vi "TimeOutPopUp.vi"(0 "Enable":bool=TRUE, 5 "error in (no error)":errorcluster, 7 "Timeout(s)":i32=2, 8 "Input Message":string="I am a Message" caption="String", 9 "Two Buttons?":bool=TRUE, 11 "Button Name":string="OK", 13 "Second Button Name":string="Cancel") -> (17 "Input":string, 18 "OK":bool, 19 "error out":errorcluster)   [LabVIEW 2018]
doc: "Displays a standard dialog box that prompts users to enter information, such as a user name and password.\n--------------------\n\nThis Express VI is configured as follows:\n\nMessage to Display to the User:I am a Message\nThe inputs are: \nText Entry Box: Input"
panel:
  out "min":dbl
  out "sec":dbl
  out "Position:Left Cancel":i32
  out "Position:Left OK1":i32
  out "Position:Top":i32
  out "Position:Left":i32
  in  "Cancel":bool
  in  "OK2":bool
  out "String":string="I am a Message" caption="There is no S11 Frequency Match. Check the Calibration and Frequency List.\nAlso Check the Frequency Units Match.\nThe test will automatically Start in 0 min 10 sec"
  in  "OK1":bool
  in  "Input 2":string caption="Input"
  out "REF":i32
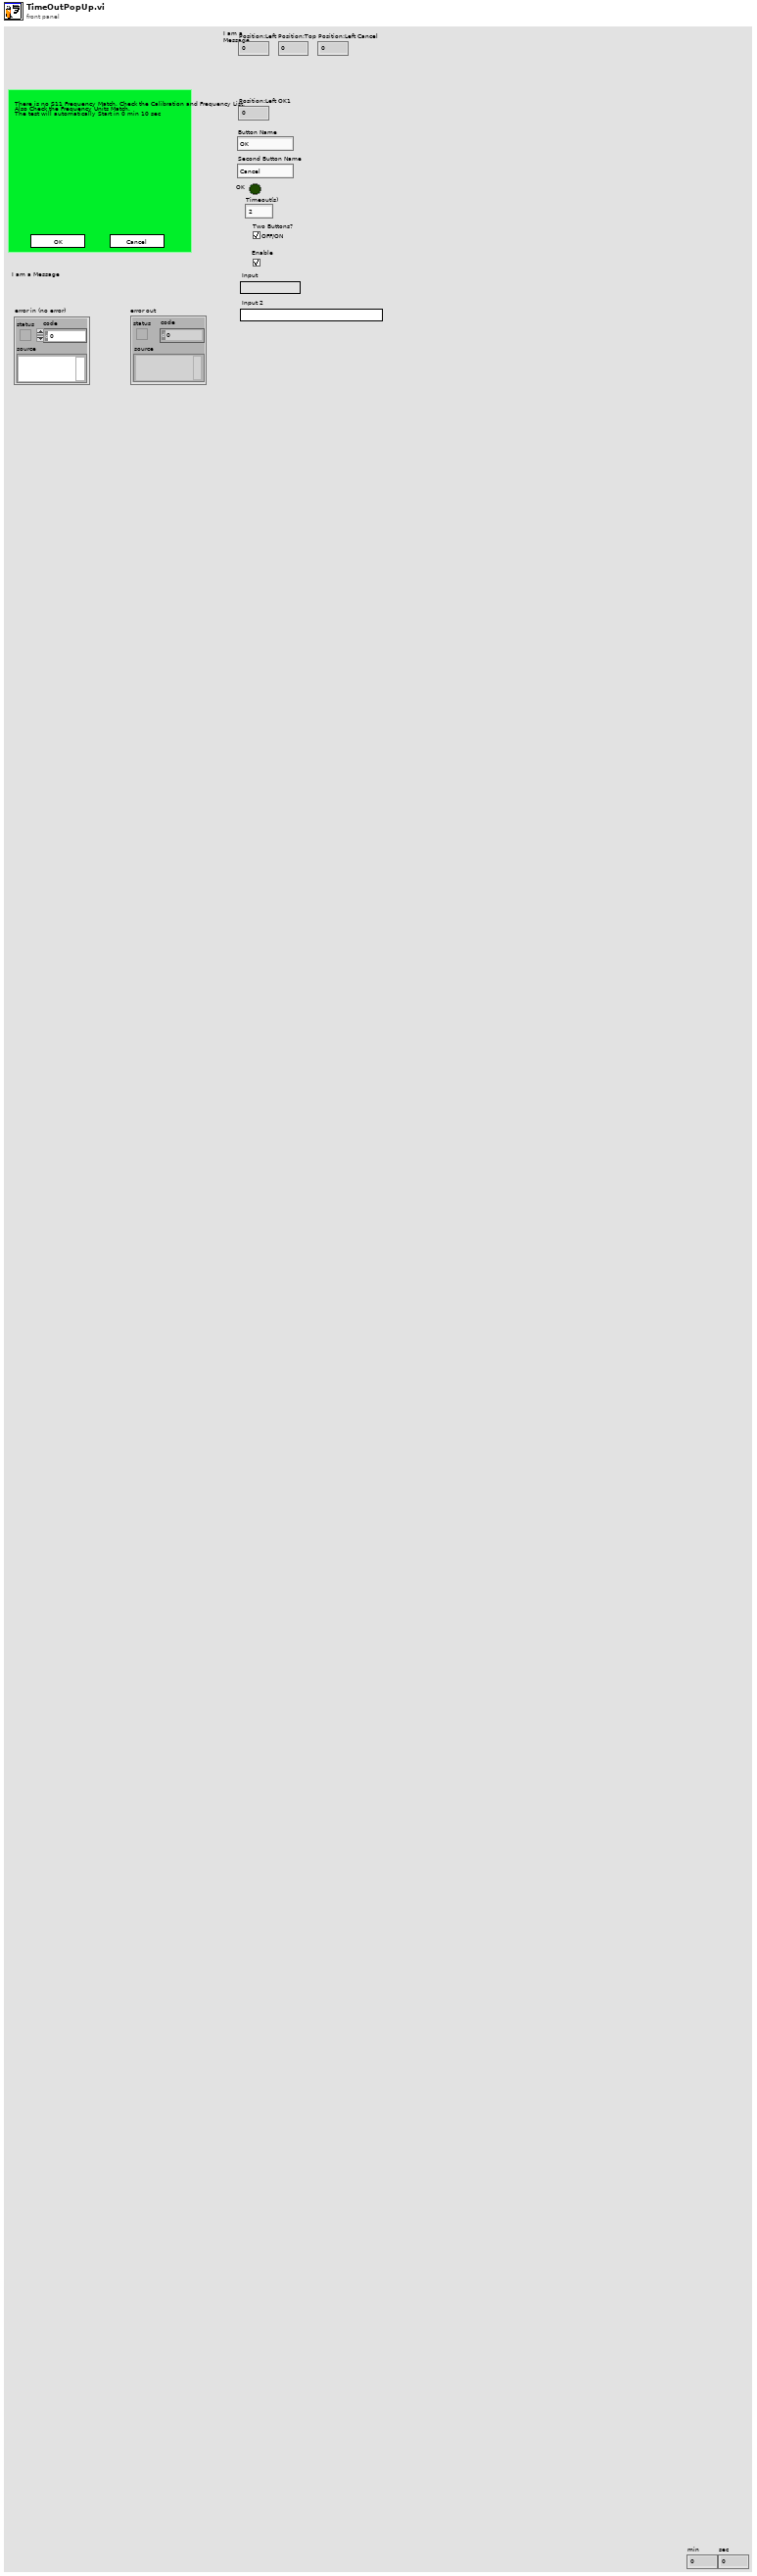
[diagram p1: front panel]
types:
  T1 = cluster{"Input Name":string, "Input Data Type":i32}[]
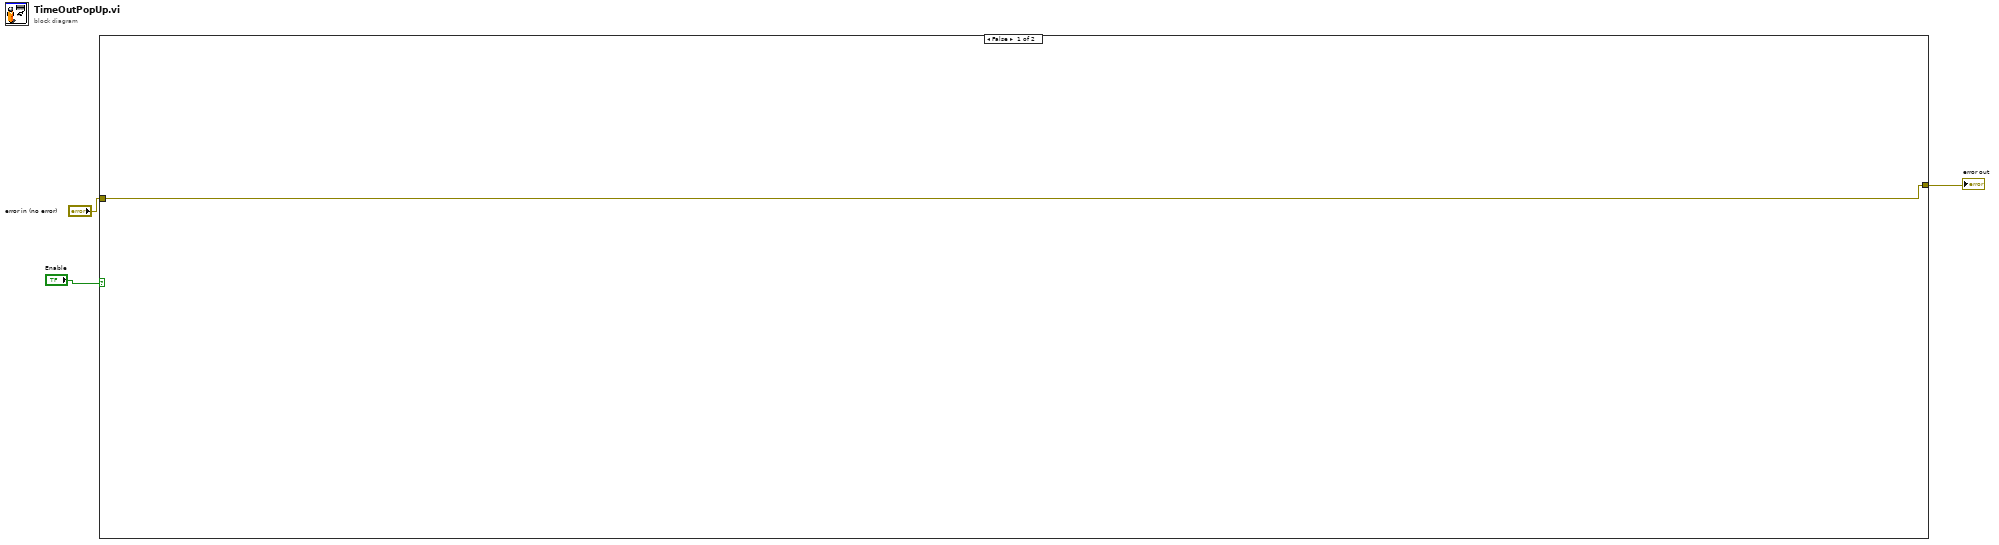
[diagram p0: block diagram]
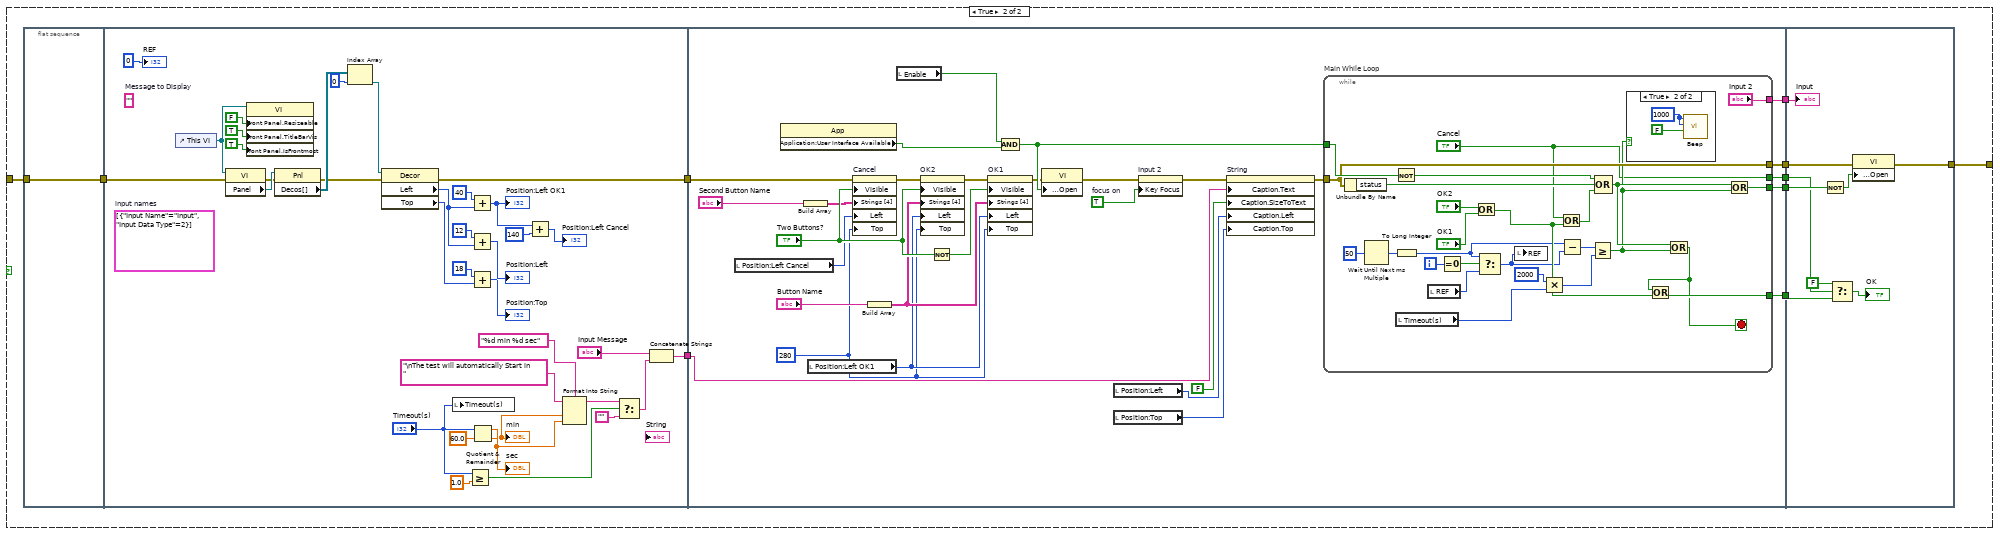
[diagram p2: hidden frame]
diagram:
  n1 = case shown="False" "Enable" {
    tunnel: "error in (no error)" -> [w4 w6]
    tunnel: [w4 w5] -> w2
    frame False {
    }
    frame True {
      n2 = flat-sequence {
        tunnel: [w15] -> w14
        tunnel: w6 -> [w15]
        tunnel: [w17] -> w13
        tunnel: [w30] -> w12
        tunnel: w14 -> [w16]
        tunnel: [w79] -> w11
        tunnel: [w75] -> w10
        tunnel: [w70] -> w9
        tunnel: [w67] -> w8
        tunnel: w13 -> [w64]
        tunnel: w12 -> [w62]
        tunnel: [w53] -> w7
        tunnel: w11 -> [w111]
        tunnel: w10 -> [w117]
        tunnel: w9 -> [w116]
        tunnel: w8 -> [w115]
        tunnel: w7 -> [w112]
        tunnel: [w109] -> w5
        frame #0 {
        }
        frame #1 {
          (unwired) T1 [{"Input Name"="Input", "Input Data Type"=2}]  # input names
          (unwired) ""  # Message to Display
          n3 = control-ref of="This VI"() -> (w35:refnum<vi>)
          n4 = property class="VI"(reference=w35, error in=w16) -> (error out=w49:errorcluster, "Panel"=w50:refnum<vi>)  [unwired: 1 out]
          n5 = property class="VI"(reference=w35, "Front Panel.Resizeable"=FALSE ("Front Panel Window:Resizable"), "Front Panel.TitleBarVis"=TRUE ("Front Panel Window:Title Bar Visible"), "Front Panel.IsFrontmost"=TRUE ("Front Panel Window:Is Frontmost")) -> ()  [unwired: 1 in, 2 out]
          n6 = property class="Pnl"(reference=w50, error in=w49) -> (error out=w31:errorcluster, "Decos[]"=w48:refnum<vi>[])  [unwired: 1 out]
          n7 = Index Array(array=w48, index=0) -> (element=w46:refnum<vi>)
          n8 = property class="Decor"(reference=w46, error in=w31) -> (error out=w30:errorcluster, "Left"=w40:i32, "Top"=w45:i32)  [unwired: 1 out]
          n9 = local write "Timeout(s)"("Timeout(s)") -> ()
          n10 = Greater Or Equal?(x="Timeout(s)", y=1.0) -> (x >= y?=w29:bool)
          n11 = Add(x=40, y=w40) -> (x+y=w37:i32)
          "Position:Left OK1" <- w37
          n12 = Add(x=12, y=w40) -> (x+y=→"Position:Left":i32)
          n13 = Add(x=18, y=w45) -> (x+y=→"Position:Top":i32)
          n14 = Quotient & Remainder(x="Timeout(s)", y=60.0) -> (x-y*floor(x/y)=w25:dbl, floor(x/y)=w24:dbl)
          "min" <- w24
          "sec" <- w25
          n15 = Add(x=w37, y=140) -> (x+y=→"Position:Left Cancel":i32)
          n16 = Format Into String(format string="%d min %d sec", initial string="\nThe test will automatically Start in " ("string"), w24, w25) -> (resulting string=w27:string)  [unwired: 1 in, 1 out]
          n17 = Select(t=w27, s=w29, f="") -> (s? t:f=w19:string)
          n18 = Concatenate Strings("Input Message", w19) -> (w17:string)
          "REF" <- u32 0 ("REF")
        }
        frame #2 {
          w54 = 280 ("Position:Top 2")
          w66 = TRUE  # focus on
          n19 = local read "Position:Left Cancel"() -> (w58:i32)
          n20 = property class="App"() -> ("Application:User Interface Available"=w68:bool)  [unwired: 2 in, 2 out]
          n21 = Build Array("Second Button Name") -> (w74:string[])
          n22 = local read "Position:Left OK1"() -> (w59:i32)
          n23 = property on="Cancel" class="Bool"(error in=w62, "Visible"="Two Buttons?", "Strings [4]"=w74, "Left"=w58, "Top"=w54) -> (error out=w77:errorcluster)  [unwired: 1 in, 1 out]
          n24 = Build Array("Button Name") -> (w72:string[])
          n25 = local read "Enable"() -> (w52:bool)
          n26 = property on="OK2" class="Bool"(error in=w77, "Visible"="Two Buttons?", "Strings [4]"=w72, "Left"=w59, "Top"=w54) -> (error out=w76:errorcluster)  [unwired: 1 in, 1 out]
          n27 = Not(x="Two Buttons?") -> (.not. x?=w78:bool)
          n28 = property on="OK1" class="Bool"(error in=w76, "Visible"=w78, "Strings [4]"=w72, "Left"=w59, "Top"=w54) -> (error out=w55:errorcluster)  [unwired: 1 in, 1 out]
          n29 = And(x=w52, y=w68) -> (x .and. y?=w69:bool)
          n30 = property class="VI"(error in=w55, "Front Panel Window:Open"=w69) -> (error out=w65:errorcluster)  [unwired: 1 in, 1 out]
          n31 = local read "Position:Left"() -> (w61:i32)
          n32 = local read "Position:Top"() -> (w60:i32)
          n33 = property on="Input 2" class="Str"(error in=w65, "Key Focus"=w66) -> (error out=w57:errorcluster)  [unwired: 1 in, 1 out]
          n34 = property on="String" class="Str"(error in=w57, "Caption.Text"=w64, "Caption.SizeToText"=FALSE ("Text.Size to Text?"), "Caption.Left"=w61, "Caption.Top"=w60) -> (error out=w56:errorcluster)  [unwired: 1 in, 1 out]
          n35 = while "Main While Loop" {
            tunnel: [w83] -> w79
            tunnel: w69 -> [w102]
            tunnel: [w87] -> w75
            tunnel: w56 -> [w99]
            tunnel: [w99] -> w70
            tunnel: ["Input 2"] -> w67
            tunnel: ["Cancel"] -> w53
            i -> [w94]
            stop <- w82 stop-if-true
            n36 = Unbundle By Name(w99) -> ("status"=w97:bool)
            n37 = Wait Until Next ms Multiple(millisecond multiple=u32 50) -> (millisecond timer value=w92:u32)
            n38 = Not(x=w102) -> (.not. x?=w101:bool)
            n39 = To Long Integer(number=w92) -> (32bit integer=w85:i32)
            n40 = local read "Timeout(s)"() -> (w86:i32)
            n41 = local read "REF"() -> (w95:i32)
            n42 = Equal To 0?(x=w94) -> (x = 0?=w93:bool)
            n43 = Or(x="OK2", y="OK1") -> (x .or. y?=w104:bool)
            n44 = Select(t=w85, s=w93, f=w95) -> (s? t:f=w91:i32)
            n45 = local write "REF"(w91) -> ()
            n46 = Multiply(x=2000, y=w86) -> (x*y=w89:i32)
            n47 = Or(x="Cancel", y=w104) -> (x .or. y?=w98:bool)
            n48 = Subtract(x=w85, y=w91) -> (x-y=w90:i32)
            n49 = Greater Or Equal?(x=w90, y=w89) -> (x >= y?=w84:bool)
            n50 = Compound Arithmetic op=OR(w101, w97, w98) -> (w100:bool)
            n51 = case shown="True" w84 {
              frame False {
              }
              frame True {
                w108 = u32 1000 ("duration (msec)")
                n52 = call <vilib>:"Beep.vi"("use system alert? (T)"=FALSE, "duration (msec)"=w108, "frequency (Hz)"=w108) -> ()  [unwired: 9 in]
              }
            }
            n53 = Or(x=w100, y=w84) -> (x .or. y?=w82:bool)
            n54 = Or(x=w82, y=w104) -> (x .or. y?=w83:bool)
            n55 = Or(x=w100, y=w84) -> (x .or. y?=w87:bool)
          }
        }
        frame #3 {
          n56 = Not(x=w117) -> (.not. x?=w114:bool)
          n57 = Select(t=FALSE, s=w112, f=w111) -> (s? t:f=→"OK":bool)
          n58 = property class="VI"(error in=w116, "Front Panel Window:Open"=w114) -> (error out=w109:errorcluster)  [unwired: 1 in, 1 out]
          "Input" <- w115
        }
      }
    }
  }
  "error out" <- w2
